vi "Setting SMU Sweeping.vi"(0 "VISA session":refnum<visa-resource-name>, 5 "Unit To Setup":u16(ring) items=["SMU 1", "SMU2", "SMU3", "SMU4", "SMU5", "SMU6", "VSU1", "VSU2"], 7 "SMU - Sweeping":T1={"Start / Offset"=0.0, "Stop / Ratio"=1.0, "Step (linear only)"=0.01, "Compliance"=0.1, "Power Compliance"=0.0, "Mode"=0, "Function"=0, "Sweep Mode"=FALSE} caption="SMU" {"Function" items=["Disabled", "Var 1", "Var 2", "Var 1'", "Constant"]; "Mode" items=["V", "I", "V pulse", "I  pulse", "Common"]; "Power Compliance" format="%^.2e"; "Compliance" format="%^.2e"; "Step (linear only)" format="%^.4e"; "Stop / Ratio" format="%^.4e"; "Start / Offset" format="%^.4e"}, 9 "Sweep spacing":u16(ring) items=["linear", "log 10", "log 25", "log 50"], 11 "Error in":errorcluster) -> (15 "Error out":errorcluster)   [LabVIEW 2014]
uses:
  <instrlib>/Agilent 415X Series/Agilent 415X Series.lvlib
panel:
  # "LICENSED MATERIALS – PROPERTY OF IBM\nCopyright IBM Corp. 2016,\nALL RIGHTS RESERVED"
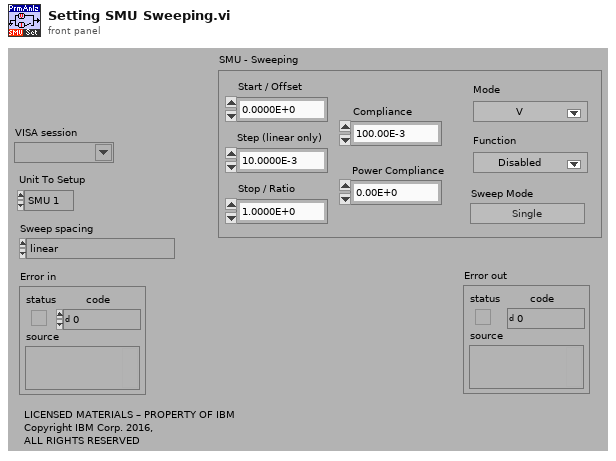
[diagram p1: front panel]
types:
  T1 = cluster{"Start / Offset":dbl, "Stop / Ratio":dbl, "Step (linear only)":dbl, "Compliance":dbl, "Power Compliance":dbl, "Mode":u32, "Function":i32, "Sweep Mode":bool}
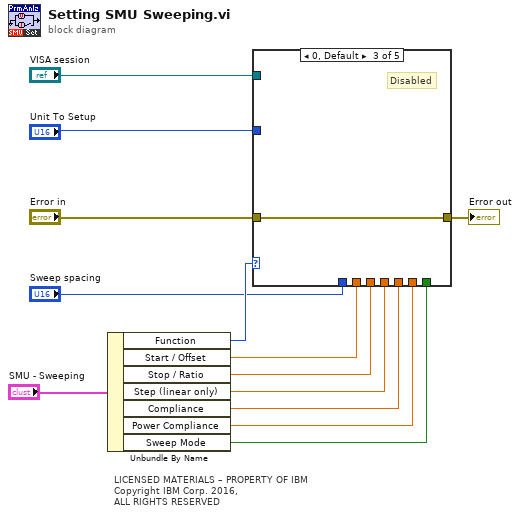
[diagram p0: block diagram]
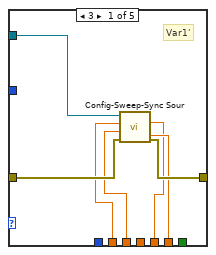
[diagram p2: hidden frame]
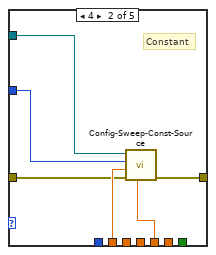
[diagram p3: hidden frame]
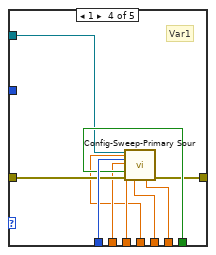
[diagram p4: hidden frame]
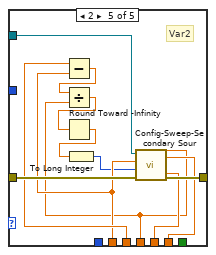
[diagram p5: hidden frame]
diagram:
  # "LICENSED MATERIALS – PROPERTY OF IBM\nCopyright IBM Corp. 2016,\nALL RIGHTS RESERVED"
  n1 = Unbundle By Name("SMU - Sweeping") -> ("Function"=w7:i32, "Start / Offset"=w13:dbl, "Stop / Ratio"=w8:dbl, "Step (linear only)"=w9:dbl, "Compliance"=w10:dbl, "Power Compliance"=w11:dbl, "Sweep Mode"=w12:bool)
  n2 = case shown="0, Default" w7 {
    tunnel: "Sweep spacing" -> [_ _ _ w37 _]
    tunnel: "Error in" -> [w20 w22 w27 w36 w48]
    tunnel: w12 -> [_ _ _ w35 _]
    tunnel: w13 -> [w15 w24 _ w34 w42]
    tunnel: w8 -> [w14 _ _ w33 w43]
    tunnel: w9 -> [_ _ _ w32 w39]
    tunnel: w10 -> [w16 w23 _ w31 w46]
    tunnel: w11 -> [w17 _ _ w30 w45]
    tunnel: [w19 w26 w27 w29 w47] -> w2
    tunnel: "VISA session" -> [w18 w25 _ w28 w49]
    tunnel: "Unit To Setup" -> [_ w21 _ _ _]
    frame 3 {
      # "Var1'"
      n3 = call <instrlib>:"Config-Sweep-Sync Sour.vi"("power compliance (0 = OFF)"=w17, "compliance"=w16, "error in (no error)"=w20, "ratio"=w14, "offset"=w15, "VISA session"=w18) -> ("error out"=w19:errorcluster)  [unwired: 5 out]
    }
    frame 4 {
      # "Constant"
      n4 = call <instrlib>:"Config-Sweep-Const-Source.vi"("compliance (SMUs only)"=w23, "error in (no error)"=w22, "source (V or A)"=w24, "unit (SMU1:0)"=w21, "VISA session"=w25) -> ("error out"=w26:errorcluster)  [unwired: 6 out]
    }
    frame 0, Default {
      # "Disabled"
    }
    frame 1 {
      # "Var1"
      n5 = call <instrlib>:"Config-Sweep-Primary Sour.vi"("VISA session"=w28, "stop"=w33, "start"=w34, "sweep spacing (linear: 0)"=w37, "step (linear only)"=w32, "sweep mode"=w35, "error in (no error)"=w36, "compliance"=w31, "power compliance (0 = OFF)"=w30) -> ("error out"=w29:errorcluster)  [unwired: 6 out]
    }
    frame 2 {
      # "Var2"
      n6 = Subtract(x=w43, y=w42) -> (x-y=w44:dbl)
      n7 = Divide(x=w44, y=w39) -> (x/y=w41:dbl)
      n8 = Round Toward -Infinity(1:w41) -> (0:w40:dbl)
      n9 = To Long Integer(number=w40) -> (32bit integer=w38:i32)
      n10 = call <instrlib>:"Config-Sweep-Secondary Sour.vi"("power compliance (0 = OFF)"=w45, "compliance"=w46, "step"=w39, "error in (no error)"=w48, "total points"=w38, "start"=w42, "VISA session"=w49) -> ("error out"=w47:errorcluster)  [unwired: 4 out]
    }
  }
  "Error out" <- w2
